vi "Configure.vi"(8 "error in (no error)":errorcluster, 11 "Build Package Item in":refnum<class "VIPM Item.lvclass">) -> (0 "error out":errorcluster, 3 "Build Package Item out":refnum<class "VIPM Item.lvclass">)   [LabVIEW 2019, in "VIPM.lvlib" / "VIPM Item.lvclass"]
uses:
  VIPM Item.lvclass
  VIPM Item.lvclass/VIPM Item.ctl
panel:
  in  "File":path
  in  "OK":bool
  in  "Cancel":bool
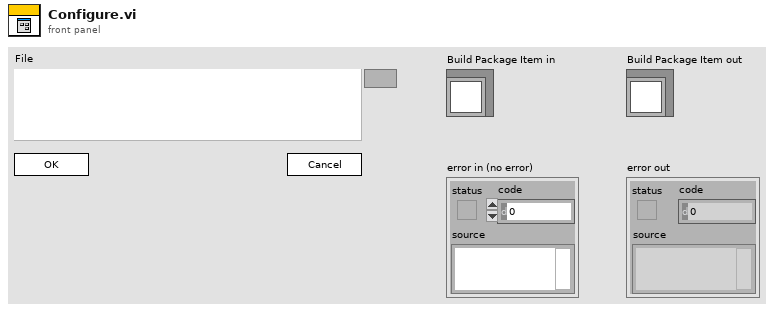
[diagram p1: front panel]
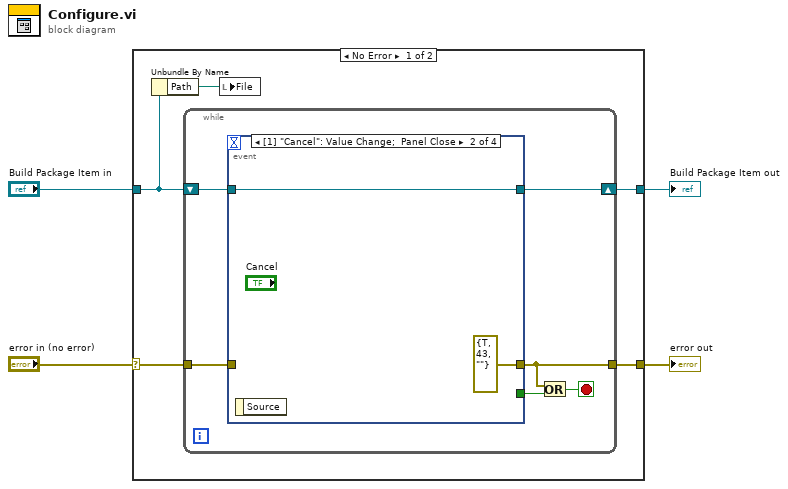
[diagram p0: block diagram]
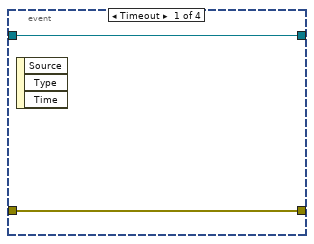
[diagram p2: hidden frame]
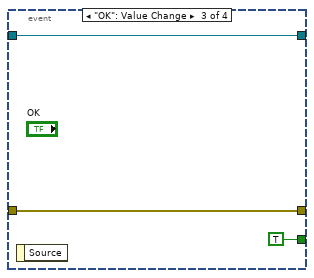
[diagram p3: hidden frame]
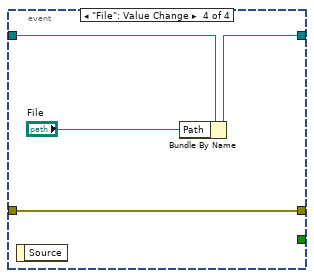
[diagram p4: hidden frame]
diagram:
  n1 = case shown="No Error" "error in (no error)" {
    selector: "error in (no error)" -> [w5 w28]
    tunnel: [w6 w28] -> w3
    tunnel: [w9 w27] -> w1
    tunnel: "Build Package Item in" -> [w8 w27]
    frame No Error {
      n2 = Unbundle By Name(w8) -> ("Path"=w7:path)
      n3 = while {
        shift-right: [w15] -> w9
        shift-left: w8 -> [w14]
        tunnel: w5 -> [w13]
        tunnel: [w11] -> w6
        stop <- w12 stop-if-true
        n4 = event shown="[1] \"Cancel\": Value Change;  Panel Close" {
          selector: _ -> [_ _ _ _]
          dyn-events: _ -> [_ _ _ _]
          timeout: _ -> [_ _ _ _]
          tunnel: w14 -> [w17 w19 w22 w26]
          tunnel: [w17 w19 w22 w25] -> w15
          tunnel: [w16 errorcluster {"status"=TRUE, "code"=43, "source"=""} ("error in (no error)") w21 w23] -> w11
          tunnel: w13 -> [w16 _ w21 w23]
          tunnel: [_ _ TRUE _] -> w10
          event Timeout {
            n5 = event-data() -> ()  [unwired: 1 in, 3 out]
          }
          event "Cancel": Value Change; Panel Close {
            n6 = event-data() -> ()  [unwired: 1 in, 1 out]
          }
          event "OK": Value Change {
            n7 = event-data() -> ()  [unwired: 1 in, 1 out]
          }
          event "File": Value Change {
            n8 = event-data() -> ()  [unwired: 1 in, 1 out]
            n9 = Bundle By Name(cluster=w26, "Path"="File") -> (w25:refnum<class "VIPM Item.lvclass">)
          }
        }
        n10 = Or(x=w11, y=w10) -> (x .or. y?=w12:bool)
      }
      n11 = local write "File"(w7) -> ()
    }
    frame Error {
    }
  }
  "error out" <- w3
  "Build Package Item out" <- w1
